vi "Stop Core.vi"(10 "final error code":i32, 11 "Stage in":refnum<class "Stage.lvclass">) -> (3 "Stage out":refnum<class "Stage.lvclass">)   [LabVIEW 2020]
doc: "(<B>Filename</B>: Actor Framework.lvlib:Actor.lvclass:Stop Core.vi)\n\nDefines what the actor does before it stops. Use the <B>final error code</B> input to determine whether the actor shut down in response to an error.\n\nBy default, this method passes the Stop message along to all auto-stop nested actors. A descendant class may override this method to define additional behavior, such as shutting down any processes the actor initiated in its override of the Actor Core method."
uses:
  <vilib>/ActorFramework/Stop Msg/Stop Msg.lvclass
  Stage.lvclass
  E:/Development/DevHardSoftware/MicroscopyFramework/Model/Hardware Abstraction Layer/Component/Device/Device/Device.lvclass
  C:/Program Files/National Instruments/LabVIEW 2020/vi.lib/ActorFramework/Actor/Actor.lvclass
  E:/Development/DevHardSoftware/MicroscopyFramework/Model/Hardware Abstraction Layer/Component/Stage/Stage/Stage.lvclass
  <vilib>/ActorFramework/Message Enqueuer/Message Enqueuer.lvclass
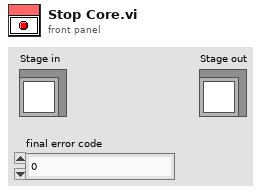
[diagram p1: front panel]
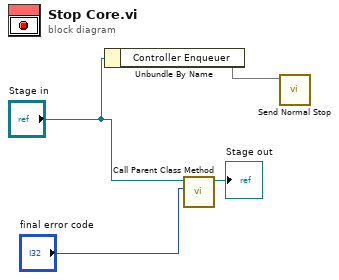
[diagram p0: block diagram]
diagram:
  n1 = Unbundle By Name("Stage in") -> ("Controller Enqueuer"=w1)
  n2 = call-parent "Call Parent Class Method"("final error code"="final error code", "Device in"="Stage in") -> ("Device out"=→"Stage out":refnum<class "Stage.lvclass">)  [unwired: 9 in]
  n3 = call <vilib>:"Send Normal Stop.vi"("Message Enqueuer"=w1) -> ()  [unwired: 10 in, 1 out]
